vi "Actor Core.vi"(8 "error in":errorcluster, 11 "GarphView In":refnum<class "GarphView.lvclass">) -> (0 "error out":errorcluster, 3 "Actor out":refnum<class "Actor.lvclass">)   [LabVIEW 2020, in "GarphView.lvlib" / "GarphView.lvclass"]
uses:
  GarphView.lvclass
  C:/Program Files (x86)/National Instruments/LabVIEW 2020/vi.lib/gpm_packages/@cs/mva-viewable/Source/IViewable/IViewable/IViewable.lvclass
  C:/Program Files (x86)/National Instruments/LabVIEW 2020/vi.lib/gpm_packages/@cs/mva-viewable/Source/ActorEvents/IEventAggregator/IEventAggregator.lvclass
  <vilib>/ActorFramework/Actor/Actor.lvclass
  <vilib>/event_ctls.llb/lveventtype.ctl
  GarphView.lvclass/GarphView.ctl
  <vilib>/gpm_packages/@cs/mva-viewable/Source/IViewable/IViewable/IViewable.lvclass
  <vilib>/gpm_packages/@cs/mva-viewable/Source/ActorEvents/IEventAggregator/IEventAggregator.lvclass
  C:/Program Files (x86)/National Instruments/LabVIEW 2020/vi.lib/gpm_packages/@cs/mva-core/Source/IObserver/IObserver/IObserver.lvclass
  C:/Program Files (x86)/National Instruments/LabVIEW 2020/vi.lib/ActorFramework/Actor/Actor.lvclass
  C:/Users/Fred Guo/Desktop/GarphTools/GarphView/GarphView/GarphView.lvclass
  <vilib>/gpm_packages/@cs/mva-viewable/Source/ActorEvents/IEventFilter/IEventFilter.lvclass
  GarphEventFilter/GarphEventFilter.lvclass
  C:/Program Files (x86)/National Instruments/LabVIEW 2020/vi.lib/gpm_packages/@cs/mva-viewable/Source/ActorEvents/IEventFilter/IEventFilter.lvclass
  C:/Users/Fred Guo/Desktop/GarphTools/GarphView/GarphEventFilter/GarphEventFilter.lvclass
panel:
  out "XY Graph":cluster{dbl[], dbl[]}[](graph) caption="XY Graph - Light"
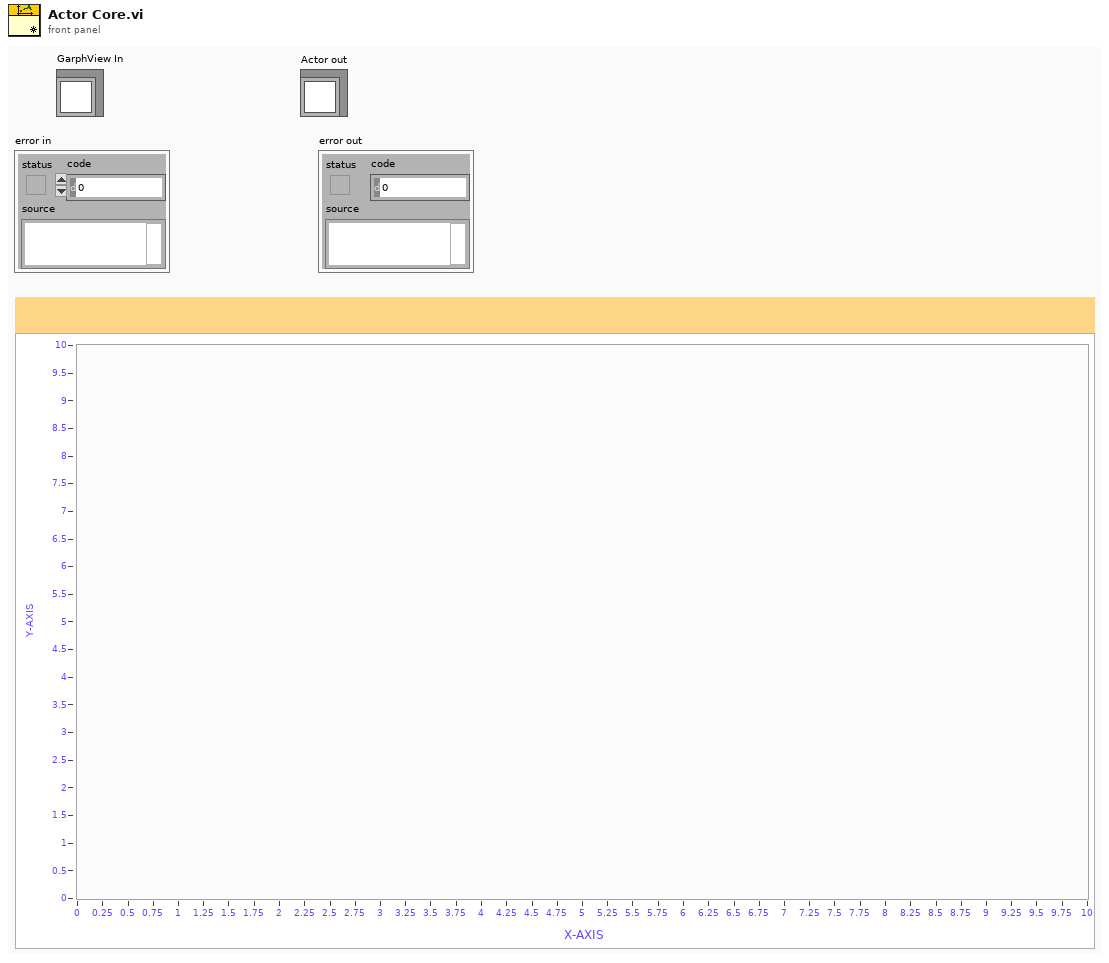
[diagram p1: front panel]
types:
  T1 = typedef "lveventtype.ctl" = enum32{"Null", "Timeout", "Annotation Menu Selection", "Annotation Menu Selection?", "App Instance Close", "App Instance Close?", "Autoscale Range Change", "Bookmark Info Change", "Cell Edit", "Cell Edit?", "Cursor Grab", "Cursor Grab?", "Cursor Menu Selection", "Cursor Menu Selection?", "Cursor Move", "Cursor Release", "Data Change", "Direction Change", "Display State Change", "Drag Ended", "Drag Enter", "Drag Leave", "Drag Over", "Drag Source Update", "Drag Starting", "Drag Starting?", "Drop", "Exec State Change", "Key Down", "Key Down?", "Key Repeat", "Key Repeat?", "Key Up", "Listbox Double Click", "Menu Activation?", "Menu Selection (App)", "Menu Selection? (App)", "Menu Selection (User)", "Mouse Down", "Mouse Down?", "Mouse Enter", "Mouse Leave", "Mouse Move", "Mouse Up", "Mouse Wheel", "NI Security User Change (App)", "Pane Size", "Panel Close", "Panel Close?", "Panel Resize", "Plot Attribute Change", "Scale Range Change", "Shortcut Menu Activation?", "Shortcut Menu Selection (App)", "Shortcut Menu Selection? (App)", "Shortcut Menu Selection (User)", "Tree Double Click", "Tree Drag", "Tree Drag?", "Tree Drop", "Tree Drop?", "Tree Item Close", "Tree Item Close?", "Tree Item Open", "Tree Item Open?", "User Event", "Value Change"}
  T2 = typedef "ActorEvents.lvlib/IEventFilter.lvclass/EventFilter Reference.ctl" = refnum<data-value>
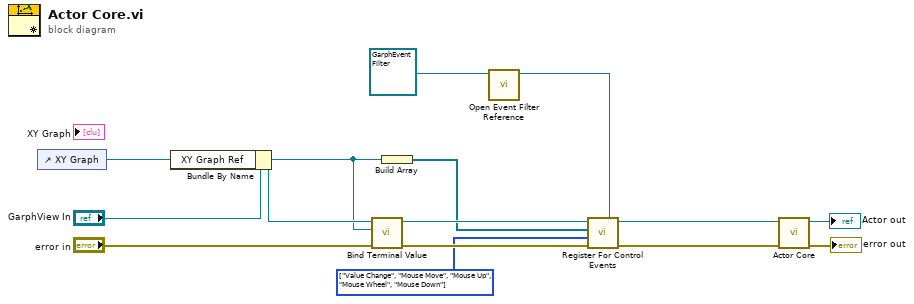
[diagram p0: block diagram]
diagram:
  w3 = T1[] [enum."Value Change", enum."Mouse Move", enum."Mouse Up", enum."Mouse Wheel", enum."Mouse Down"] items=["Null", "Timeout", "Annotation Menu Selection", "Annotation Menu Selection?", "App Instance Close", "App Instance Close?", "Autoscale Range Change", "Bookmark Info Change", "Cell Edit", "Cell Edit?", "Cursor Grab", "Cursor Grab?", "Cursor Menu Selection", "Cursor Menu Selection?", "Cursor Move", "Cursor Release", "Data Change", "Direction Change", "Display State Change", "Drag Ended", "Drag Enter", "Drag Leave", "Drag Over", "Drag Source Update", "Drag Starting", "Drag Starting?", "Drop", "Exec State Change", "Key Down", "Key Down?", "Key Repeat", "Key Repeat?", "Key Up", "Listbox Double Click", "Menu Activation?", "Menu Selection (App)", "Menu Selection? (App)", "Menu Selection (User)", "Mouse Down", "Mouse Down?", "Mouse Enter", "Mouse Leave", "Mouse Move", "Mouse Up", "Mouse Wheel", "NI Security User Change (App)", "Pane Size", "Panel Close", "Panel Close?", "Panel Resize", "Plot Attribute Change", "Scale Range Change", "Shortcut Menu Activation?", "Shortcut Menu Selection (App)", "Shortcut Menu Selection? (App)", "Shortcut Menu Selection (User)", "Tree Double Click", "Tree Drag", "Tree Drag?", "Tree Drop", "Tree Drop?", "Tree Item Close", "Tree Item Close?", "Tree Item Open", "Tree Item Open?", "User Event", "Value Change"] ("Registration Types")
  n1 = control-ref of="XY Graph"() -> (w5:refnum<vi>)
  n2 = Bundle By Name(cluster="GarphView In", "XY Graph Ref"=w5) -> (w11:refnum<class "GarphView.lvclass">)
  n3 = call <vilib>:"Bind Terminal Value.vi"("error in (no error)"="error in", "Ctl Refnum"=w5, "IViewable in"=w11) -> ("error out"=w7:errorcluster, "IViewable out"=w9:refnum<class "GarphView.lvclass">)  [unwired: 7 in]
  n4 = Build Array(w5) -> (w4:refnum<vi>[])
  n5 = call <vilib>:"Open Event Filter Reference.vi"("IEventFilter in"=refnum<class "GarphEventFilter.lvclass"> refnum ("GarphView.lvlib:GarphEventFilter.lvclass")) -> ("IEventFilter Reference"=w1:T2)  [unwired: 9 in, 1 out]
  n6 = call <vilib>:"Register For Control Events.vi"("EventFilter Reference"=w1, "error in (no error)"=w7, "Registration Types"=w3, "Control Refnums"=w4, "IEventAggregator In"=w9) -> ("error out"=w6:errorcluster, "IEventAggregator Out"=w8:refnum<class "GarphView.lvclass">)  [unwired: 5 in]
  n7 = call-parent "Actor Core.vi"("error in"=w6, "IViewable In"=w8) -> ("error out"=→"error out":errorcluster, "Actor out"=→"Actor out":refnum<class "Actor.lvclass">)  [unwired: 8 in]
